vi "Discovery Loop Async.vi"(11 "DiscoveryService in":refnum<class "DiscoveryService.lvclass">) -> ()   [LabVIEW 2020, in "Vecto.lvlib" / "DiscoveryService.lvclass"]
uses:
  DiscoveryService.lvclass
  DiscoveryService.lvclass/DiscoveryService.ctl
  proto/Discovery/Class/Msg.lvclass/Msg.ctl
  proto/Discovery/Class/Msg.lvclass
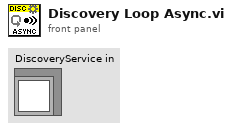
[diagram p1: front panel]
types:
  T1 = typedef "Service.lvlib/Data.ctl" = cluster{"type":T2, "port":i32}
  T2 = typedef "ServiceType.lvlib/Enumeration.ctl" = enum16{"SERVICETYPE_UNKNOWN", "SERVICETYPE_TCPSERVER", "SERVICETYPE_HTTPSERVER"}
  T3 = typedef "Discovery.lvlib/Data.ctl" = cluster{"node_id":u32, "name":string, "ip":u32, "status":string, "services":T1[], "system":string, "cluster":string}
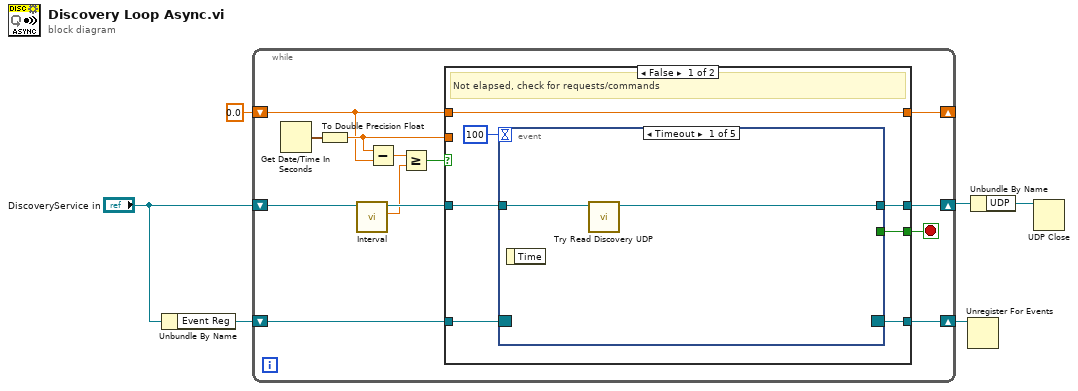
[diagram p0: block diagram]
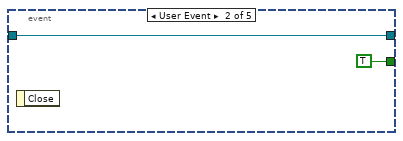
[diagram p2: hidden frame]
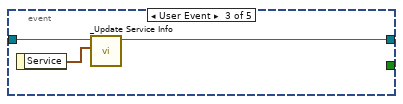
[diagram p3: hidden frame]
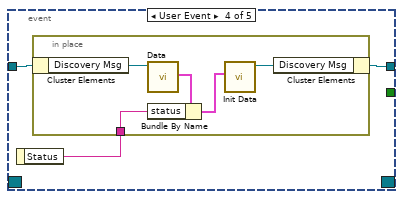
[diagram p4: hidden frame]
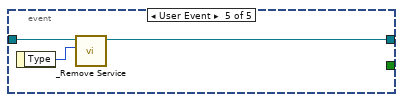
[diagram p5: hidden frame]
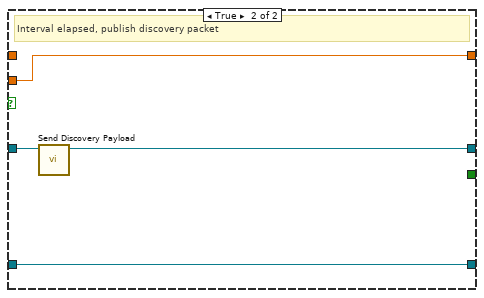
[diagram p6: hidden frame]
diagram:
  n1 = Unbundle By Name("DiscoveryService in") -> ("Event Reg"=w4:refnum<event-registration>)
  n2 = while {
    shift-right: [w13] -> _
    shift-left: 0.0 -> [w15]
    shift-right: [w12] -> w2
    shift-left: "DiscoveryService in" -> [w17]
    shift-right: [w10] -> w3
    shift-left: w4 -> [w11]
    stop <- w9 stop-if-true
    n3 = Get Date/Time In Seconds() -> (seconds since 1Jan1904=w19:timestamp)
    n4 = To Double Precision Float(number=w19) -> (double precision float=w16:dbl)
    n5 = call "Interval.vi"("DiscoveryService in"=w17) -> ("Interval S"=w7:dbl, "DiscoveryService out"=w8:refnum<class "DiscoveryService.lvclass">)  [unwired: 8 in, 1 out]
    n6 = Subtract(x=w16, y=w15) -> (x-y=w18:dbl)
    n7 = Greater Or Equal?(x=w18, y=w7) -> (x >= y?=w14:bool)
    n8 = case shown="False" w14 {
      tunnel: w8 -> [w24 w47]
      tunnel: w16 -> [_ w48]
      tunnel: w15 -> [w26 _]
      tunnel: [w26 w48] -> w13
      tunnel: [w23 w46] -> w12
      tunnel: w11 -> [w22 w45]
      tunnel: [w21 w45] -> w10
      tunnel: [w20 _] -> w9
      frame False {
        # "Not elapsed, check for requests/commands"
        n9 = event shown="[0] Timeout" {
          selector: w22 -> [_ _ _ _ _]
          dyn-events: [_ _ _ _ _] -> w21
          timeout: 100 -> [_ _ _ _ _]
          tunnel: w24 -> [w28 w30 w33 w36 w44]
          tunnel: [w27 w30 w31 w34 w42] -> w23
          tunnel: [_ TRUE _ _ _] -> w20
          event Timeout {
            n10 = event-data() -> ()  [unwired: 1 in, 1 out]
            n11 = call "Try Read Discovery UDP.vi"("DiscoveryService in"=w28) -> ("DiscoveryService out"=w27:refnum<class "DiscoveryService.lvclass">)  [unwired: 9 in, 1 out]
          }
          event User Event {
            n12 = event-data() -> ()  [unwired: 1 in, 1 out]
          }
          event User Event {
            n13 = event-data() -> ("Service"=w32:T1)  [unwired: 1 in]
            n14 = call "_Update Service Info.vi"("Service"=w32, "DiscoveryService in"=w33) -> ("DiscoveryService out"=w31:refnum<class "DiscoveryService.lvclass">)  [unwired: 8 in, 1 out]
          }
          event User Event {
            n15 = event-data() -> ("Status"=w35:string)  [unwired: 1 in]
            n16 = in-place {
              in-place-border: w35 -> [w39]
              n17 = in-place-cluster #1(w36) -> ("Discovery Msg"=w41:refnum<class "Msg.lvclass">)
              n18 = call "Data.vi"("PB Msg Template in"=w41) -> ("Data"=w40:T3)  [unwired: 8 in, 2 out]
              n19 = Bundle By Name(cluster=w40, "status"=w39) -> (w38:T3)
              n20 = call "Init Data.vi"("Data"=w38) -> ("Msg out"=w37:refnum<class "Msg.lvclass">)  [unwired: 10 in]
              n21 = in-place-cluster #1("Discovery Msg"=w37) -> (w34:refnum<class "DiscoveryService.lvclass">)
            }
          }
          event User Event {
            n22 = event-data() -> ("Type"=w43:T2)  [unwired: 1 in]
            n23 = call "_Remove Service.vi"("Type"=w43, "DiscoveryService in"=w44) -> ("DiscoveryService out"=w42:refnum<class "DiscoveryService.lvclass">)  [unwired: 8 in, 1 out]
          }
        }
      }
      frame True {
        # "Interval elapsed, publish discovery packet"
        n24 = call "Send Discovery Payload.vi"("DiscoveryService in"=w47) -> ("DiscoveryService out"=w46:refnum<class "DiscoveryService.lvclass">)  [unwired: 9 in, 1 out]
      }
    }
  }
  n25 = Unregister For Events(event registration refnum=w3) -> ()  [unwired: 1 in, 1 out]
  n26 = Unbundle By Name(w2) -> ("UDP"=w1:refnum<k16>)
  n27 = UDP Close(connection ID=w1) -> ()  [unwired: 1 in, 2 out]
